vi "Demo1.vi"   [LabVIEW 2012]
types:
  T1 = typedef "BotSpeak_Control.ctl" = cluster{"Address":string, "Reply EOF":string, "Hardware":path, "Retries":i8, "Timeout":i32}
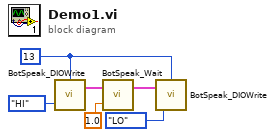
[diagram p0: block diagram]
diagram:
  w4 = u8 13 ("Port")
  n1 = call <userlib>:"BotSpeak_DIOWrite.vi"("State"=enum32{"LO", "HI"}."HI", "DIO Line"=w4) -> ("Bot Settings"=w6:T1)  [unwired: 1 in, 1 out]
  n2 = call <userlib>:"BotSpeak_Wait.vi"("Wait (sec)"=sgl 1.0 ("delay (s)"), "Bot Settings"=w6) -> ("Bot Settings"=w5:T1)  [unwired: 1 in]
  n3 = call <userlib>:"BotSpeak_DIOWrite.vi"("State"=enum32{"LO", "HI"}."LO", "Bot Settings"=w5, "DIO Line"=w4) -> ()  [unwired: 2 out]
